vi "Connect to Server.vi"(8 "error in (no error)":errorcluster, 11 "WebSocket Client in":refnum<class "WebSocket Client.lvclass">) -> (0 "error out":errorcluster, 3 "WebSocket Client out":refnum<class "WebSocket Client.lvclass">)   [LabVIEW 2021, in "WebSockets.lvlib" / "WebSocket Client.lvclass"]
doc: "Opens a conenction and creates a new WebSocket Client using the NI VISA TCP Socket.\nWebSockets 2.0.1.40\nSam Sharp - MediaMongrels Ltd\nCopyright (c) 2019, MediaMongrels Ltd"
uses:
  WebSocket Client.lvclass
  D:/my_projects/projects/Algorithms/Labview/21/WebSockets/Source/WebSockets/WebSocket/WebSocket.lvclass
  WebSocket/WebSocket.lvclass/WebSocket.ctl
  WebSocket/Read Socket.vi
  WebSocket/Write Socket.vi
  WebSocket/Read read operation timeout.vi
  Sockets/Socket/Socket.lvclass
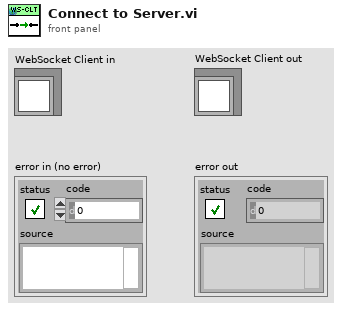
[diagram p1: front panel]
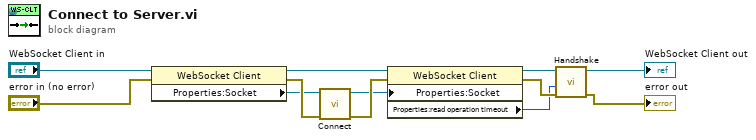
[diagram p0: block diagram]
diagram:
  n1 = property class="WebSocket Client"(reference="WebSocket Client in", error in="error in (no error)") -> (reference out=w7:refnum<class "WebSocket Client.lvclass">, error out=w10:errorcluster, "Properties:Socket"=w9:refnum<class "Socket.lvclass">)
  n2 = call-dynamic "Connect.vi"("error in (no error)"=w10, "Socket in"=w9) -> ("error out"=w8:errorcluster, "Socket out"=w2:refnum<class "Socket.lvclass">)  [unwired: 8 in]
  n3 = property class="WebSocket Client"(reference=w7, error in=w8, "Properties:Socket"=w2) -> (reference out=w5:refnum<class "WebSocket Client.lvclass">, error out=w6:errorcluster, "Properties:read operation timeout"=w1:i32)
  n4 = call-dynamic "Handshake.vi"("error in (no error)"=w6, "timeout ms (5000)"=w1, "WebSocket Client in"=w5) -> ("error out"=→"error out":errorcluster, "WebSocket Client out"=→"WebSocket Client out":refnum<class "WebSocket Client.lvclass">)  [unwired: 7 in]
